vi "Read Keyboard.vi"() -> (1 "forwardOrReverse":dbl, 2 "leftOrRight":dbl)   [LabVIEW 2018]
uses:
  Global Teleop Variables.vi
  <vilib>/Utility/inputDevices.llb/keyboardAcquire.vi
panel:
  out "element":T1(ring)
  out "keys pressed":T2(array[ring])
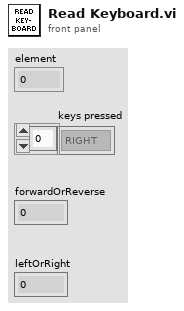
[diagram p1: front panel]
types:
  T1 = enum16{"0", "1", "2", "3", "4", "5", "6", "7", "8", "9", "A", "B", "C", "D", "E", "F", "G", "H", "I", "J", "K", "L", "M", "N", "O", "P", "Q", "R", "S", "T", "U", "V", "W", "X", "Y", "Z", "F1", "F2", "F3", "F4", "F5", "F6", "F7", "F8", "F9", "F10", "F11", "F12", "F13", "F14", "F15", "ADD", "BACK", "BACKSLASH", "CAPITAL", "COMMA", "DECIMAL", "DELETE", "DIVIDE", "DOWN", "END", "EQUALS", "ESCAPE", "GRAVE (`)", "HOME", "INSERT", "LBRACKET", "LCONTROL", "LEFT", "L ALT", "LSHIFT", "LWIN", "MINUS", "MULTIPLY", "NEXT", "NUMLOCK", "NUMPAD_0", "NUMPAD_1", "NUMPAD_2", "NUMPAD_3", "NUMPAD_4", "NUMPAD_5", "NUMPAD_6", "NUMPAD_7", "NUMPAD_8", "NUMPAD_9", "PAUSE", "PERIOD", "PRIOR (PG UP)", "RBRACKET", "RCONTROL", "RETURN", "RIGHT", "R ALT", "RSHIFT", "RWIN", "SCROLL", "SEMICOLON", "SLASH", "SPACE", "SUBTRACT", "TAB", "UP", "ENTER (num pad)", "' (quote)"}
  T2 = enum16{"0", "1", "2", "3", "4", "5", "6", "7", "8", "9", "A", "B", "C", "D", "E", "F", "G", "H", "I", "J", "K", "L", "M", "N", "O", "P", "Q", "R", "S", "T", "U", "V", "W", "X", "Y", "Z", "F1", "F2", "F3", "F4", "F5", "F6", "F7", "F8", "F9", "F10", "F11", "F12", "F13", "F14", "F15", "ADD", "BACK", "BACKSLASH", "CAPITAL", "COMMA", "DECIMAL", "DELETE", "DIVIDE", "DOWN", "END", "EQUALS", "ESCAPE", "GRAVE (`)", "HOME", "INSERT", "LBRACKET", "LCONTROL", "LEFT", "L ALT", "LSHIFT", "LWIN", "MINUS", "MULTIPLY", "NEXT", "NUMLOCK", "NUMPAD_0", "NUMPAD_1", "NUMPAD_2", "NUMPAD_3", "NUMPAD_4", "NUMPAD_5", "NUMPAD_6", "NUMPAD_7", "NUMPAD_8", "NUMPAD_9", "PAUSE", "PERIOD", "PRIOR (PG UP)", "RBRACKET", "RCONTROL", "RETURN", "RIGHT", "R ALT", "RSHIFT", "RWIN", "SCROLL", "SEMICOLON", "SLASH", "SPACE", "SUBTRACT", "TAB", "UP", "ENTER (num pad)", "' (quote)"}[]
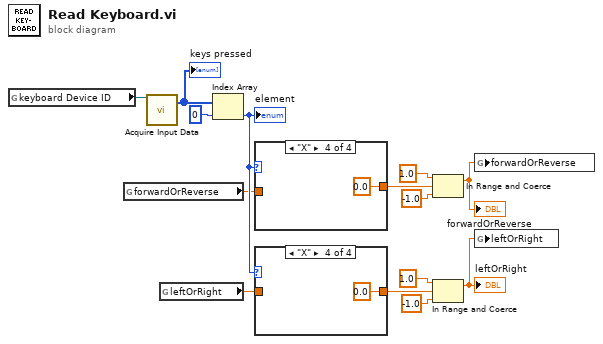
[diagram p0: block diagram]
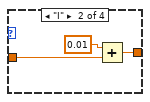
[diagram p3: hidden frame]
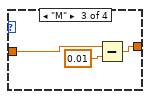
[diagram p4: hidden frame]
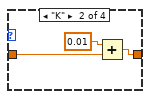
[diagram p6: hidden frame]
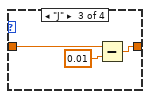
[diagram p7: hidden frame]
diagram:
  n1 = global read "Global Teleop Variables.vi" "keyboard Device ID"() -> (w5:refnum<k1>)
  n2 = global read "Global Teleop Variables.vi" "forwardOrReverse"() -> (w12:dbl)
  n3 = call-poly <vilib>:"Acquire Input Data.vi"("device ID"=w5) -> ("keys pressed"=w3:T2)  [unwired: 16 in, 2 out]
  "keys pressed" <- w3
  n4 = global read "Global Teleop Variables.vi" "leftOrRight"() -> (w6:dbl)
  n5 = Index Array(array=w3, index=0) -> (element=w13:T1)
  "element" <- w13
  n6 = case shown="\"X\"" w13 {
    tunnel: w12 -> [w15 w17 w20 _]
    tunnel: [w15 w16 w19 0.0 ("forwardOrReverse")] -> w14
    frame "0", Default {
    }
    frame "I" {
      n7 = Add(x=0.01, y=w17) -> (x+y=w16:dbl)
    }
    frame "M" {
      n8 = Subtract(x=w20, y=0.01) -> (x-y=w19:dbl)
    }
    frame "X" {
    }
  }
  n9 = case shown="\"X\"" w13 {
    tunnel: [w23 w25 w27 0.0 ("leftOrRight")] -> w9
    tunnel: w6 -> [w23 w24 w29 _]
    frame "0", Default {
    }
    frame "K" {
      n10 = Add(x=0.01, y=w24) -> (x+y=w25:dbl)
    }
    frame "J" {
      n11 = Subtract(x=w29, y=0.01) -> (x-y=w27:dbl)
    }
    frame "X" {
    }
  }
  n12 = In Range and Coerce(upper limit=1.0, x=w14, lower limit=-1.0) -> (coerced(x)=w2:dbl)  [unwired: 1 out]
  "forwardOrReverse" <- w2
  n13 = In Range and Coerce(upper limit=1.0, x=w9, lower limit=-1.0) -> (coerced(x)=w1:dbl)  [unwired: 1 out]
  "leftOrRight" <- w1
  n14 = global write "Global Teleop Variables.vi" "forwardOrReverse"(w2) -> ()
  n15 = global write "Global Teleop Variables.vi" "leftOrRight"(w1) -> ()
